vi "CRYSelect New Channel.vi"(10 "Channel In":T1, 11 "Channel Name In":string) -> (0 "Change":bool, 1 "Status":string, 3 "Channel Name  Out":string)   [LabVIEW 2013]
uses:
  CRYSystem/Typedef Control/CRYChanged Data Array Cluster.ctl
  CRYSystem/Typedef Control/CRYChanged Data Cluster.ctl
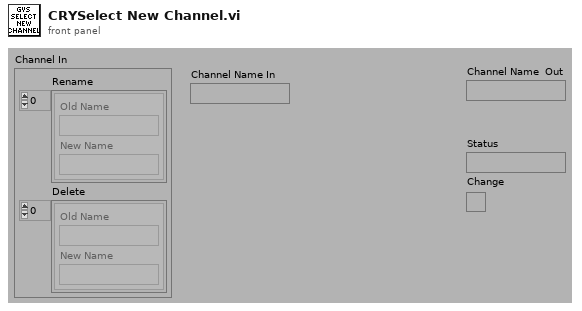
[diagram p1: front panel]
types:
  T1 = typedef "CRYChanged Data Array Cluster.ctl" = cluster{"Rename":T2[], "Delete":T2[]}
  T2 = typedef "CRYChanged Data Cluster.ctl" = cluster{"Old Name":string, "New Name":string}
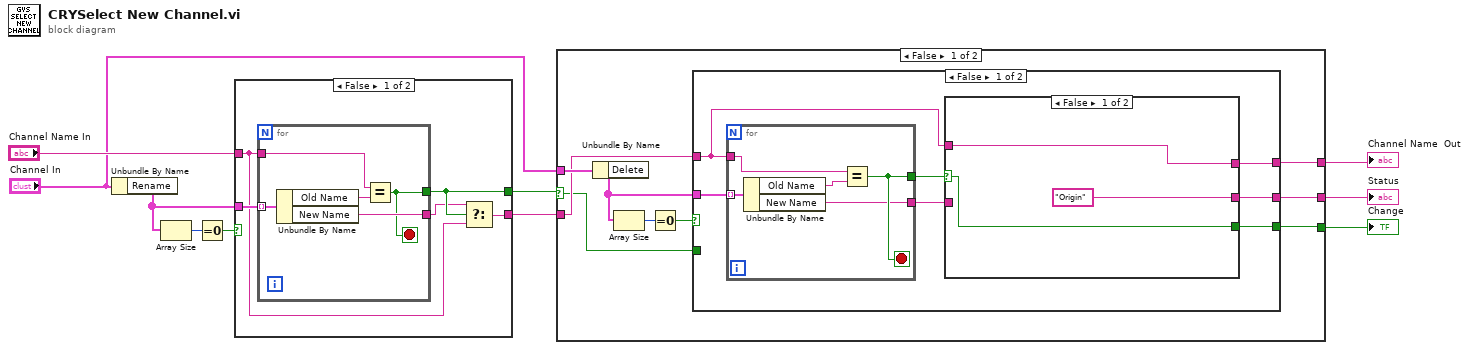
[diagram p0: block diagram]
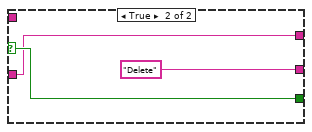
[diagram p2: hidden frame]
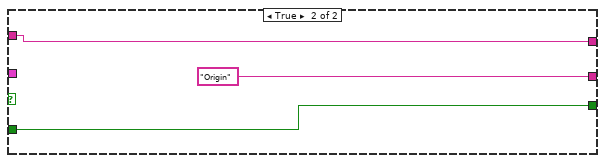
[diagram p3: hidden frame]
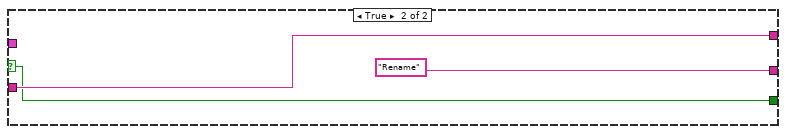
[diagram p4: hidden frame]
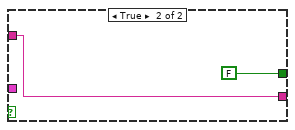
[diagram p5: hidden frame]
diagram:
  n1 = Unbundle By Name("Channel In") -> ("Rename"=w7:T2[])
  n2 = Array Size(array=w7) -> (size(s)=w8:i32)
  n3 = Equal To 0?(x=w8) -> (x = 0?=w6:bool)
  n4 = case shown="False" w6 {
    tunnel: w7 -> [w15 _]
    tunnel: "Channel Name In" -> [w12 w21]
    tunnel: [w11 w21] -> w5
    tunnel: [w14 FALSE] -> w4
    frame False {
      n5 = for {
        tunnel: w15 -> [w20] mode=indexing
        tunnel: w12 -> [w18]
        tunnel: [w17] -> w13
        tunnel: [w16] -> w14
        stop <- w16 stop-if-true
        n6 = Unbundle By Name(w20) -> ("Old Name"=w19:string, "New Name"=w17:string)
        n7 = Equal?(x=w18, y=w19) -> (x = y?=w16:bool)
      }
      n8 = Select(t=w13, s=w14, f=w12) -> (s? t:f=w11:string)
    }
    frame True {
    }
  }
  n9 = case shown="False" w4 {
    selector: w4 -> [w24 w54]
    tunnel: [w26 w55] -> w9
    tunnel: w5 -> [w27 w55]
    tunnel: "Channel In" -> [w28 _]
    tunnel: [w25 w54] -> w3
    tunnel: [w23 "Rename" ("Status")] -> w1
    frame False {
      n10 = Unbundle By Name(w28) -> ("Delete"=w31:T2[])
      n11 = Array Size(array=w31) -> (size(s)=w29:i32)
      n12 = Equal To 0?(x=w29) -> (x = 0?=w30:bool)
      n13 = case shown="False" w30 {
        tunnel: w31 -> [w34 _]
        tunnel: w27 -> [w36 w52]
        tunnel: [w37 w52] -> w26
        tunnel: [w35 w51] -> w25
        tunnel: w24 -> [_ w51]
        tunnel: [w32 "Origin"] -> w23
        frame False {
          n14 = for {
            tunnel: w36 -> [w48]
            tunnel: w34 -> [w49] mode=indexing
            tunnel: [w46] -> w38
            tunnel: [w45] -> w33
            stop <- w46 stop-if-true
            n15 = Unbundle By Name(w49) -> ("Old Name"=w47:string, "New Name"=w45:string)
            n16 = Equal?(x=w48, y=w47) -> (x = y?=w46:bool)
          }
          n17 = case shown="False" w38 {
            selector: w38 -> [w40 w44]
            tunnel: [w41 w43] -> w37
            tunnel: w36 -> [w41 _]
            tunnel: [w40 w44] -> w35
            tunnel: w33 -> [_ w43]
            tunnel: ["Origin" "Delete" ("Status")] -> w32
            frame False {
            }
            frame True {
            }
          }
        }
        frame True {
        }
      }
    }
    frame True {
    }
  }
  "Channel Name  Out" <- w9
  "Change" <- w3
  "Status" <- w1
